vi "ActionVIOnCompile.vi"(8 "error in":errorcluster, 11 "Device Item Ref in":T16=18446744073709551615) -> (0 "error out":errorcluster)   [LabVIEW 2019, in "Fuel Injector Analysis Addon System Explorer.lvlib"]
uses:
  Fuel Injector Analysis Addon System Explorer.lvlib
  <vilib>/NI VeriStand/Custom Device API/Custom Device Item Ref.ctl
  Addon Shared/Types/Compiled.Settings.ctl
  Addon Shared/Types/Injector info.ctl
  Addon Shared/Types/Compiled.Group.WaveformRefs.ctl
  <vilib>/NI VeriStand/Custom Device API/Waveform Data Reference.ctl
  <vilib>/NI VeriStand/Custom Device API/Block Data Reference.ctl
  <vilib>/NI VeriStand/Custom Device API/Data Reference.ctl
  Addon Shared/Types/VS.Register.Info.ctl
  Addon Shared/Types/Register.Info.ctl
  Addon Shared/Types/FPGA Data Types.ctl
  Addon Shared/Types/Compiled.Group.Timing.ctl
  Addon Shared/Types/Shot.Parameters.ctl
  Addon Shared/Types/Stage.Parameters.ctl
  Addon Shared/Types/Stage.PullIn.Types.ctl
  Addon Shared/Types/Stage.Transition.Types.ctl
  Addon Shared/Types/Analysis.Channels.Select.ctl
  <vilib>/NI VeriStand/Custom Device API/Data Access Type.ctl
  <vilib>/NI VeriStand/Custom Device API/Custom Device Target Type.ctl
  Addon Shared/SubVIs/Constants.vi
  <vilib>/NI VeriStand/Custom Device Tools/Custom Device Utility Library/NI VeriStand - Search for Item by GUID.vi
  <vilib>/NI VeriStand/Custom Device Tools/Custom Device Utility Library/NI VeriStand - Search for All Items by GUID.vi
  <vilib>/NI VeriStand/Custom Device Tools/Custom Device Utility Library/NI VeriStand - Search for Item by Name.vi
  <vilib>/NI VeriStand/Custom Device API/Get Item Property (Double).vi
  <vilib>/NI VeriStand/Custom Device API/Get Item Property (U32).vi
  <vilib>/NI VeriStand/Custom Device API/Set Item Property (Variant).vi
  Addon Shared/Fuel Injector Analysis Addon Shared.lvlib
  <vilib>/NI VeriStand/Custom Device API/Custom Device API.lvlib
  <vilib>/NI VeriStand/Custom Device Tools/Custom Device Utility Library/Custom Device Utility Library.lvlib
  <vilib>/NI/NIVS Inline Async API/_Data Access System Explorer/Data Access System Explorer.lvlib
panel:
  out "output cluster":T1={"Name"="", "RIO.Address"="", "Bitfile.Path"=path "", "Injectors.Count"=0, "Injectors.Settings"=[], "Waveform.Refs"=[], "VS.Registers"={"Block Data refs"=[], "Values"=[]}, "Registers"=[], "Timing.Registers"=[], "Mux.Register"={"Name"="", "Data Type"=enum."<Null>", "Default Value"=variant(dbl 0.0)}, "Groups.Settings"=[]} {"Mux.Register"."Data Type" format="%.0x"; "Registers"."Register"."Data Type" format="%.0x"; "VS.Registers"."Block Data refs"."Data Reference" format="%.0x"}
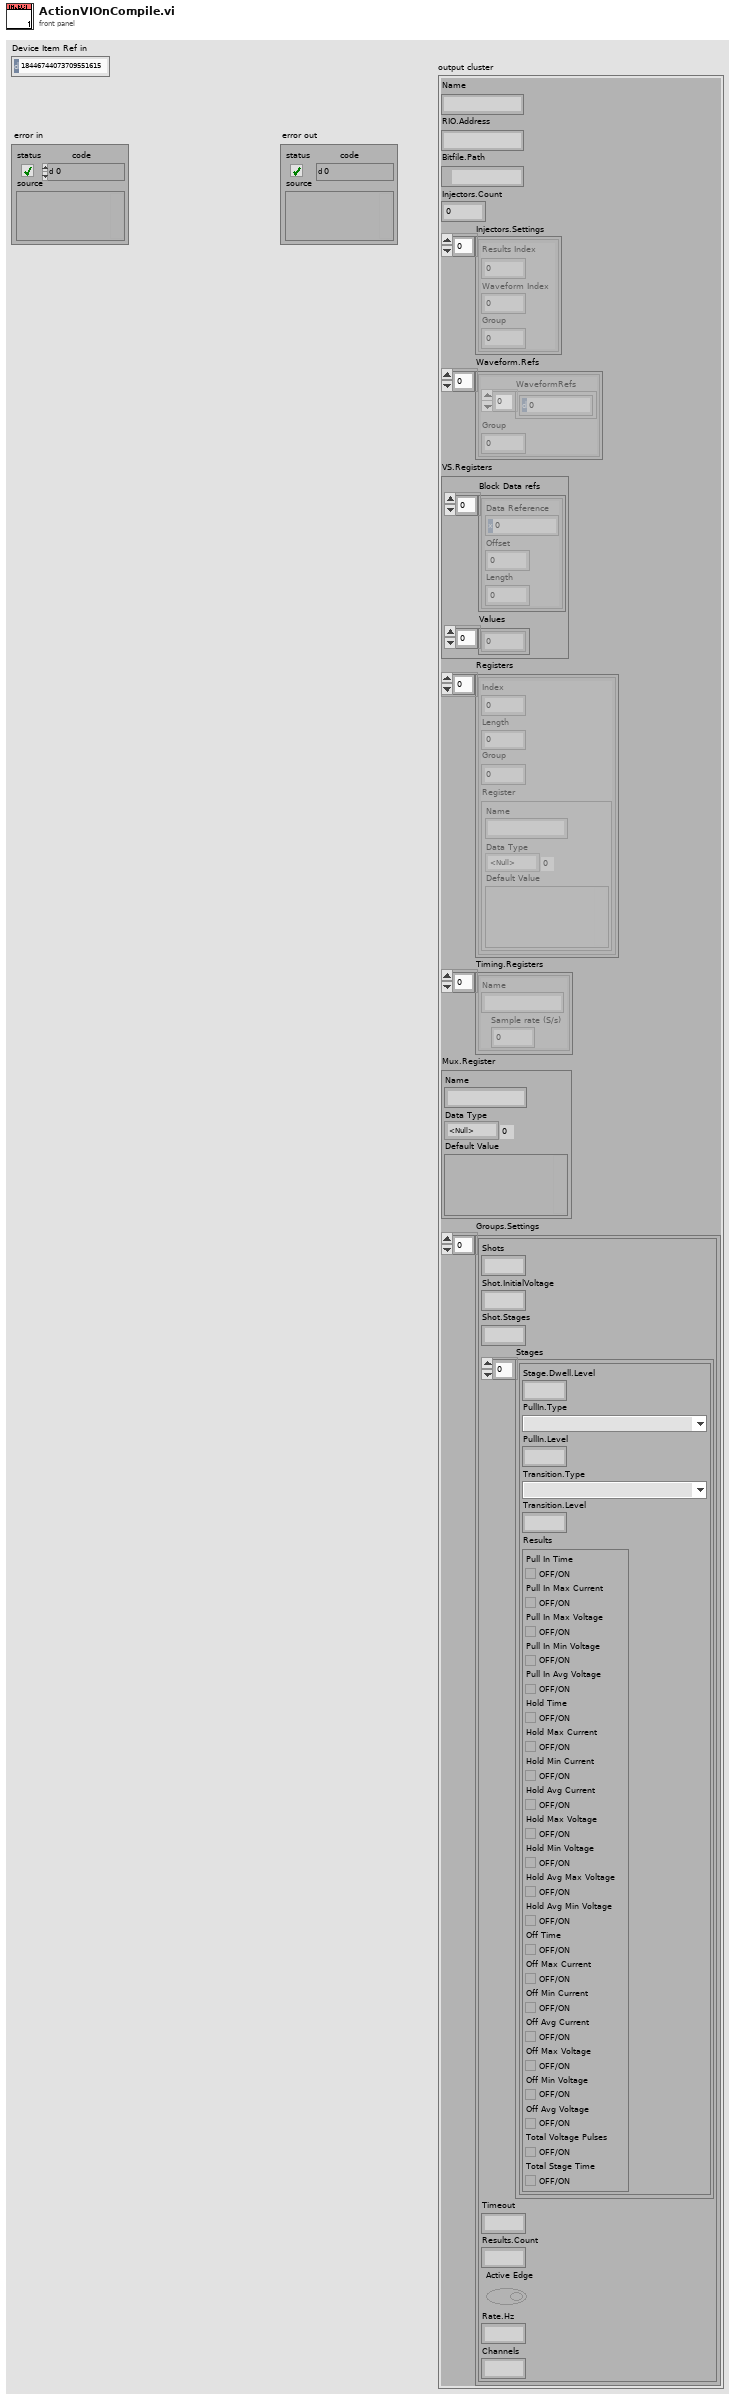
[diagram p1: front panel]
types:
  T1 = typedef "Fuel Injector Analysis Addon Shared.lvlib/Compiled.Settings.ctl" = cluster{"Name":string, "RIO.Address":string, "Bitfile.Path":path, "Injectors.Count":u32, "Injectors.Settings":T2[], "Waveform.Refs":T3[], "VS.Registers":cluster{"Block Data refs":T5[], "Values":dbl[]}, "Registers":T7[], "Timing.Registers":T10[], "Mux.Register":T8, "Groups.Settings":T11[]}
  T2 = typedef "Fuel Injector Analysis Addon Shared.lvlib/Injector info.ctl" = cluster{"Results Index":i32, "Waveform Index":i32, "Group":u16}
  T3 = typedef "Fuel Injector Analysis Addon Shared.lvlib/Compiled.Group.WaveformRefs.ctl" = cluster{"WaveformRefs":T4[], "Group":i32}
  T4 = typedef "Custom Device API.lvlib/Waveform Data Reference.ctl" = i32
  T5 = typedef "Custom Device API.lvlib/Block Data Reference.ctl" = cluster{"Data Reference":T6, "Offset":u64, "Length":u64}
  T6 = typedef "Custom Device API.lvlib/Data Reference.ctl" = i32
  T7 = typedef "Fuel Injector Analysis Addon Shared.lvlib/VS.Register.Info.ctl" = cluster{"Index":i32, "Length":i32, "Group":i32, "Register":T8}
  T8 = typedef "Fuel Injector Analysis Addon Shared.lvlib/Register.Info.ctl" = cluster{"Name":string, "Data Type":T9, "Default Value":variant}
  T9 = typedef "Fuel Injector Analysis Addon Shared.lvlib/FPGA Data Types.ctl" = enum8{"<Null>", "Injector.Core.Setting", "Injector.Global.Setting", "Injector.Mux.Setting", "Injector.Timing"}
  T10 = typedef "Fuel Injector Analysis Addon Shared.lvlib/Compiled.Group.Timing.ctl" = cluster{"Name":string, "Sample rate (S/s)":u32}
  T11 = typedef "Fuel Injector Analysis Addon Shared.lvlib/Shot.Parameters.ctl" = cluster{"Shots":u32, "Shot.InitialVoltage":dbl, "Shot.Stages":u32, "Stages":T12[], "Timeout":dbl, "Results.Count":i32, "Active Edge":bool, "Rate.Hz":u32, "Channels":u32}
  T12 = typedef "Fuel Injector Analysis Addon Shared.lvlib/Stage.Parameters.ctl" = cluster{"Stage.Dwell.Level":dbl, "PullIn.Type":T13, "PullIn.Level":dbl, "Transition.Type":T14, "Transition.Level":dbl, "Results":T15}
  T13 = typedef "Fuel Injector Analysis Addon Shared.lvlib/Stage.PullIn.Types.ctl" = enum8{"Pull In Transition Pulses", "Pull In Transition Current Drop"}
  T14 = typedef "Fuel Injector Analysis Addon Shared.lvlib/Stage.Transition.Types.ctl" = enum8{"Stage Transition Inactive Time", "Stage Transition Voltage Increase", "Stage Transition Current Decrease", "Stage Transition Active Time"}
  T15 = typedef "Fuel Injector Analysis Addon Shared.lvlib/Analysis.Channels.Select.ctl" = cluster{"Pull In Time":bool, "Pull In Max Current":bool, "Pull In Max Voltage":bool, "Pull In Min Voltage":bool, "Pull In Avg Voltage":bool, "Hold Time":bool, "Hold Max Current":bool, "Hold Min Current":bool, "Hold Avg Current":bool, "Hold Max Voltage":bool, "Hold Min Voltage":bool, "Hold Avg Max Voltage":bool, "Hold Avg Min Voltage":bool, "Off Time":bool, "Off Max Current":bool, "Off Min Current":bool, "Off Avg Current":bool, "Off Max Voltage":bool, "Off Min Voltage":bool, "Off Avg Voltage":bool, "Total Voltage Pulses":bool, "Total Stage Time":bool}
  T16 = typedef "Custom Device API.lvlib/Custom Device Item Ref.ctl" = u64
  T17 = enum16{"Output/Write", "Input/Read", "Input/ReadWrite"}
  T18 = typedef "Custom Device API.lvlib/Custom Device Target Type.ctl" = enum16{"PharLap", "VxWorks", "Windows", "Linux_32_ARM", "Linux_x64"}
  T19 = typedef "Custom Device API.lvlib/Data Access Type.ctl" = enum16{"Read", "Write"}
  T20 = cluster{"Name":string, "Type":enum16{"Output/Write", "Input/Read", "Input/ReadWrite"}, "VS Refs":T16[]}
  T21 = typedef "Custom Device API.lvlib/Custom Device Item Info.ctl" = cluster{"Name":string, "Is Channel":bool, "GUID":string, "Is Waveform":bool}
  T22 = typedef "Fuel Injector Analysis Addon Shared.lvlib/Main Settings.ctl" = cluster{"RIO Device Address":string, "Local bitfile path":path, "RT bitfile path":path, "Number of injectors":u16}
  T23 = typedef "Custom Device API.lvlib/Custom Device Channel.ctl" = cluster{"Type":T24, "Units":string, "Default Value":dbl, "Faultable":bool, "Scalable":bool}
  T24 = typedef "Custom Device API.lvlib/Custom Device Channel Type.ctl" = enum16{"Input", "Output"}
  T25 = cluster{"Name":string, "Type":enum16{"Output/Write", "Input/Read", "Input/ReadWrite"}, "VS Refs":T16[]}[]
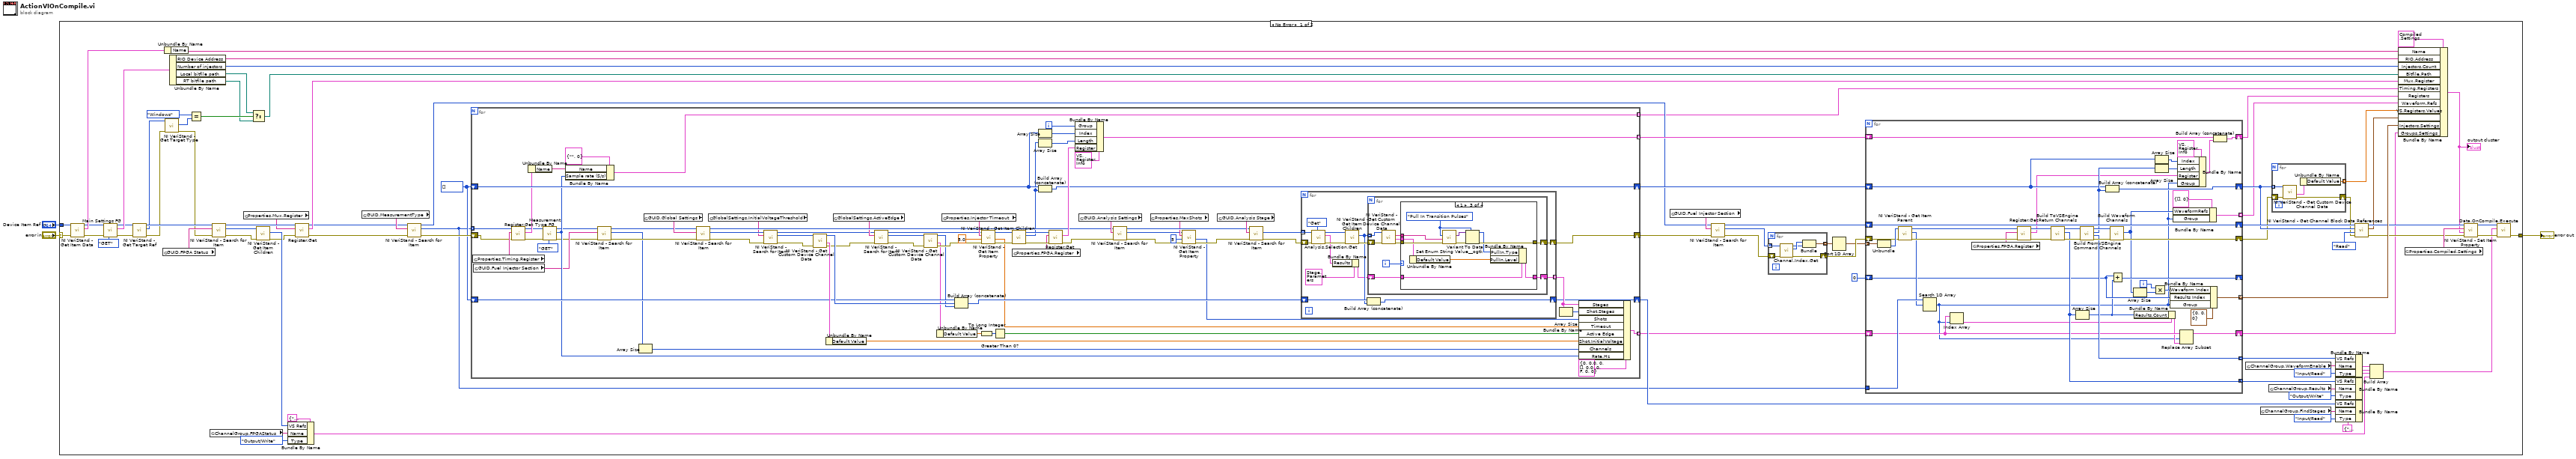
[diagram p0: block diagram]
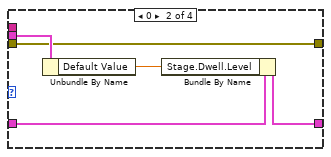
[diagram p3: hidden frame]
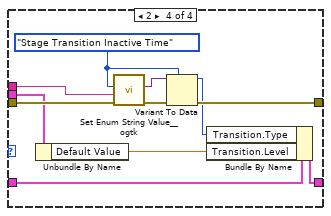
[diagram p4: hidden frame]
diagram:
  n1 = case shown="No Error" "error in" {
    selector: "error in" -> [w88 w275]
    tunnel: "Device Item Ref in" -> [w87 _]
    tunnel: [w76 w275] -> w1
    frame No Error {
      w13 = T16[] []
      w24 = T20 {"Name"="", "Type"=enum."Input/Read", "VS Refs"=[]} ("Group")
      n2 = call <vilib>:"NI VeriStand - Get Item Data.vi"("error in (no error)"=w88, "Item Ref in"=w87) -> ("error out"=w84:errorcluster, "Item Info"=w86:T21, "Item Ref out"=w83:T16)  [unwired: 6 in, 1 out]
      n3 = call "Main Settings FG.vi"("Action"=enum8{"GET", "SET"}."GET", "error in (no error)"=w84, "Item Ref"=w83) -> ("error out"=w44:errorcluster, "Main Settings out"=w82:T22, "Item Ref out"=w59:T16)  [unwired: 6 in]
      n4 = call <vilib>:"NI VeriStand - Get Target Ref.vi"("error in"=w44, "Item Ref in"=w59) -> ("error out"=w42:errorcluster, "Target Ref"=w43:T16, "Item Ref out"=w45:T16)  [unwired: 6 in, 1 out]
      n5 = global read "Constants.vi" "GUID.FPGA Status"() -> (w58:string)
      n6 = Unbundle By Name(w86) -> ("Name"=w85:string)
      n7 = call <vilib>:"NI VeriStand - Get Target Type.vi"("error in (no error)"=w42, "Item Ref in"=w43) -> ("error out"=w41:errorcluster, "Target Type"=w40:T18)  [unwired: 7 in, 1 out]
      n8 = Unbundle By Name(w82) -> ("RIO Device Address"=w81:string, "Number of injectors"=w71:u16, "Local bitfile path"=w36:path, "RT bitfile path"=w37:path)
      n9 = Equal?(x=Custom_Device_Target_Type."Windows", y=w40) -> (x = y?=w38:bool)
      n10 = global read "Constants.vi" "ChannelGroup.FPGAStatus"() -> (w55:string)
      n11 = call-poly <vilib>:"NI VeriStand - Search for Item.vi"("error in"=w41, "Item GUID"=w58, "Section Ref in"=w45) -> ("error out"=w53:errorcluster, "Item Ref"=w57:T16, "Section Ref out"=w51:T16)  [unwired: 5 in, 1 out]
      n12 = global read "Constants.vi" "Properties.Mux.Register"() -> (w49:string)
      n13 = Select(t=w36, s=w38, f=w37) -> (s? t:f=w35:path)
      n14 = call <vilib>:"NI VeriStand - Get Item Children.vi"("error in (no error)"=w53, "Item Ref in"=w57) -> ("error out"=w50:errorcluster, "Child Refs"=w54:T16[])  [unwired: 6 in, 2 out]
      n15 = Bundle By Name(cluster=T20 {"Name"="", "Type"=enum."Input/Read", "VS Refs"=[]} ("Group"), "VS Refs"=w54, "Name"=w55, "Type"=T17."Output/Write") -> (w52:T20)
      n16 = call "Register.Get.vi"("error in (no error)"=w50, "Property"=w49, "Section Ref in"=w51) -> ("error out"=w7:errorcluster, "Register"=w48:T8, "Item Ref out"=w6:T16)  [unwired: 6 in]
      n17 = global read "Constants.vi" "GUID.MeasurementType"() -> (w15:string)
      n18 = call-poly <vilib>:"NI VeriStand - Search for Item.vi"("error in"=w7, "Item GUID"=w15, "Section Ref in"=w6) -> ("error out"=w16:errorcluster, "Item Refs"=w12:T16[], "Section Ref out"=w11:T16)  [unwired: 5 in, 1 out]
      n19 = for {
        tunnel: [w126] -> w63 mode=indexing
        shift-right: [w160] -> w28
        shift-left: w16 -> [w105]
        shift-right: [w133] -> w23
        shift-left: w13 -> [w130]
        shift-right: [w124] -> w64
        shift-left: w13 -> [w128]
        tunnel: w12 -> [w104] mode=indexing
        tunnel: [w123] -> w10 mode=indexing
        tunnel: [w102] -> w5 mode=indexing
        i -> [w95]
        n20 = global read "Constants.vi" "Properties.Timing.Register"() -> (w108:string)
        n21 = global read "Constants.vi" "GUID.Fuel Injector Section"() -> (w98:string)
        n22 = call "Register.Get.vi"("error in (no error)"=w105, "Property"=w108, "Section Ref in"=w104) -> ("error out"=w94:errorcluster, "Register"=w107:T8, "Item Ref out"=w92:T16)  [unwired: 6 in]
        n23 = Unbundle By Name(w107) -> ("Name"=w106:string)
        n24 = call "Measurement Type FG.vi"("Action"=enum8{"GET", "SET"}."GET", "error in (no error)"=w94, "Item Ref"=w92) -> ("error out"=w93:errorcluster, "Sample rate (S/s)"=w101:u32, "Item Ref out"=w91:T16)  [unwired: 6 in]
        n25 = Bundle By Name(cluster=T10 {"Name"="", "Sample rate (S/s)"=0}, "Name"=w106, "Sample rate (S/s)"=w101) -> (w102:T10)
        n26 = call-poly <vilib>:"NI VeriStand - Search for Item.vi"("error in"=w93, "Item GUID"=w98, "Section Ref in"=w91) -> ("error out"=w100:errorcluster, "Item Refs"=w97:T16[], "Section Ref out"=w99:T16)  [unwired: 5 in, 1 out]
        n27 = Array Size(array=w97) -> (size(s)=w96:i32)
        n28 = global read "Constants.vi" "GUID.Global Settings"() -> (w167:string)
        n29 = call-poly <vilib>:"NI VeriStand - Search for Item.vi"("error in"=w100, "Item GUID"=w167, "Section Ref in"=w99) -> ("error out"=w141:errorcluster, "Item Ref"=w140:T16, "Section Ref out"=w149:T16)  [unwired: 5 in, 1 out]
        n30 = global read "Constants.vi" "GlobalSettings.InitialVoltageThreshold"() -> (w139:string)
        n31 = call-poly <vilib>:"NI VeriStand - Search for Item.vi"("error in"=w141, "Item Name"=w139, "Section Ref in"=w140) -> ("error out"=w136:errorcluster, "Item Ref"=w135:T16, "Section Ref out"=w118:T16)  [unwired: 5 in, 1 out]
        n32 = call <vilib>:"NI VeriStand - Get Custom Device Channel Data.vi"("error in (no error)"=w136, "Channel Ref in"=w135) -> ("error out"=w117:errorcluster, "Channel"=w137:T23, "Channel Ref out"=w134:T16)  [unwired: 4 in, 3 out]
        n33 = Unbundle By Name(w137) -> ("Default Value"=w131:dbl)
        n34 = global read "Constants.vi" "GlobalSettings.ActiveEdge"() -> (w119:string)
        n35 = call-poly <vilib>:"NI VeriStand - Search for Item.vi"("error in"=w117, "Item Name"=w119, "Section Ref in"=w118) -> ("error out"=w120:errorcluster, "Item Ref"=w121:T16, "Section Ref out"=w110:T16)  [unwired: 5 in, 1 out]
        n36 = call <vilib>:"NI VeriStand - Get Custom Device Channel Data.vi"("error in (no error)"=w120, "Channel Ref in"=w121) -> ("error out"=w116:errorcluster, "Channel"=w114:T23, "Channel Ref out"=w115:T16)  [unwired: 4 in, 3 out]
        n37 = Unbundle By Name(w114) -> ("Default Value"=w113:dbl)
        n38 = global read "Constants.vi" "Properties.Injector Timeout"() -> (w156:string)
        n39 = Build Array (concatenate)(w130, w134, w115) -> (w138:T16[])
        n40 = To Long Integer(number=w113) -> (32bit integer=w112:i32)
        n41 = call-poly <vilib>:"NI VeriStand - Get Item Property.vi"("error in (no error)"=w116, "Default Value"=5.0, "Property Name"=w156, "Item Ref in"=w110) -> ("error out"=w155:errorcluster, "Value"=w122:dbl, "Item Ref out"=w154:T16)  [unwired: 4 in, 1 out]
        n42 = Greater Than 0?(x=w112) -> (x > 0?=w111:bool)
        n43 = call <vilib>:"NI VeriStand - Get Item Children.vi"("error in (no error)"=w155, "Item Ref in"=w154) -> ("error out"=w165:errorcluster, "Child Refs"=w125:T16[], "Item Ref out"=w162:T16)  [unwired: 6 in, 1 out]
        n44 = global read "Constants.vi" "Properties.FPGA.Register"() -> (w161:string)
        n45 = Array Size(array=w128) -> (size(s)=w127:i32)
        n46 = Array Size(array=w125) -> (size(s)=w129:i32)
        n47 = Build Array (concatenate)(w128, w125) -> (w124:T16[])
        n48 = call "Register.Get.vi"("error in (no error)"=w165, "Property"=w161, "Section Ref in"=w162) -> ("error out"=w147:errorcluster, "Register"=w163:T8)  [unwired: 6 in, 1 out]
        n49 = Bundle By Name(cluster=T7 {"Index"=0, "Length"=0, "Group"=0, "Register"={"Name"="", "Data Type"=enum."<Null>", "Default Value"=variant}} ("Cluster"), "Group"=w95, "Index"=w127, "Length"=w129, "Register"=w163) -> (w126:T7)
        n50 = global read "Constants.vi" "GUID.Analysis Settings"() -> (w150:string)
        n51 = call-poly <vilib>:"NI VeriStand - Search for Item.vi"("error in"=w147, "Item GUID"=w150, "Section Ref in"=w149) -> ("error out"=w143:errorcluster, "Item Ref"=w144:T16, "Section Ref out"=w148:T16)  [unwired: 5 in, 1 out]
        n52 = global read "Constants.vi" "Properties.MaxShots"() -> (w145:string)
        n53 = call-poly <vilib>:"NI VeriStand - Get Item Property.vi"("error in (no error)"=w143, "Default Value"=u32 5, "Property Name"=w145, "Item Ref in"=w144) -> ("error out"=w142:errorcluster, "Value"=w132:u32)  [unwired: 4 in, 2 out]
        n54 = global read "Constants.vi" "GUID.Analysis Stage"() -> (w166:string)
        n55 = call-poly <vilib>:"NI VeriStand - Search for Item.vi"("error in"=w142, "Item GUID"=w166, "Section Ref in"=w148) -> ("error out"=w159:errorcluster, "Item Refs"=w158:T16[])  [unwired: 5 in, 2 out]
        n56 = for {
          tunnel: w158 -> [w180] mode=indexing
          shift-right: [w175] -> w160
          shift-left: w159 -> [w181]
          tunnel: [w174] -> w152 mode=indexing
          shift-right: [w171] -> w133
          shift-left: w138 -> [w173]
          n57 = call "Analysis.Selection.Get.vi"("Action"=enum8{"Get", "Set"}."Get", "error in (no error)"=w181, "Item Ref in"=w180) -> ("error out"=w178:errorcluster, "Selections"=w168:T15, "Item Ref out"=w176:T16)  [unwired: 6 in]
          n58 = Bundle By Name(cluster=T12 {"Stage.Dwell.Level"=0.0, "PullIn.Type"=enum."Pull In Transition Pulses", "PullIn.Level"=0.0, "Transition.Type"=enum."Stage Transition Voltage Increase", "Transition.Level"=0.0, "Results"={"Pull In Time"=TRUE, "Pull In Max Current"=TRUE, "Pull In Max Voltage"=TRUE, "Pull In Min Voltage"=TRUE, "Pull In Avg Voltage"=TRUE, "Hold Time"=TRUE, "Hold Max Current"=TRUE, "Hold Min Current"=TRUE, "Hold Avg Current"=TRUE, "Hold Max Voltage"=TRUE, "Hold Min Voltage"=TRUE, "Hold Avg Max Voltage"=TRUE, "Hold Avg Min Voltage"=TRUE, "Off Time"=TRUE, "Off Max Current"=TRUE, "Off Min Current"=TRUE, "Off Avg Current"=TRUE, "Off Max Voltage"=TRUE, "Off Min Voltage"=TRUE, "Off Avg Voltage"=TRUE, "Total Voltage Pulses"=TRUE, "Total Stage Time"=TRUE}}, "Results"=w168) -> (w169:T12)
          n59 = call <vilib>:"NI VeriStand - Get Item Children.vi"("error in (no error)"=w178, "Item Ref in"=w176) -> ("error out"=w177:errorcluster, "Child Refs"=w172:T16[])  [unwired: 6 in, 2 out]
          n60 = Build Array (concatenate)(w173, w172) -> (w171:T16[])
          n61 = for {
            shift-right: [w184] -> w175
            shift-left: w177 -> [w190]
            tunnel: w172 -> [w189] mode=indexing
            shift-right: [w182] -> w174
            shift-left: w169 -> [w183]
            i -> [w187]
            n62 = call <vilib>:"NI VeriStand - Get Custom Device Channel Data.vi"("error in (no error)"=w190, "Channel Ref in"=w189) -> ("error out"=w188:errorcluster, "Channel"=w186:T23, "Channel Name"=w185:string)  [unwired: 4 in, 3 out]
            n63 = case shown="1" w187 {
              tunnel: w188 -> [w192 w196 w208 w219]
              tunnel: w186 -> [_ w197 w203 w213]
              tunnel: w185 -> [_ _ w207 w218]
              tunnel: [w192 w196 w202 w214] -> w184
              tunnel: w183 -> [w191 w195 w201 w211]
              tunnel: [w191 w193 w200 w210] -> w182
              frame Default {
              }
              frame 0 {
                n64 = Unbundle By Name(w197) -> ("Default Value"=w194:dbl)
                n65 = Bundle By Name(cluster=w195, "Stage.Dwell.Level"=w194) -> (w193:T12)
              }
              frame 1 {
                w204 = Stage.PullIn.Types."Pull In Transition Pulses" ("PullIn.Type")
                n66 = Unbundle By Name(w203) -> ("Default Value"=w198:dbl)
                n67 = call <userlib>:"Set Enum String Value__ogtk.vi"("error in (no error)"=w208, "String Value"=w207, "Default Enum Value"=w204) -> ("error out"=w206:errorcluster, "Enum"=w205:variant)  [unwired: 7 in]
                n68 = Variant To Data(error in=w206, type=w204, Variant=w205) -> (data=w199:T13, error out=w202:errorcluster)
                n69 = Bundle By Name(cluster=w201, "PullIn.Type"=w199, "PullIn.Level"=w198) -> (w200:T12)
              }
              frame 2 {
                w215 = Stage.Transition.Types."Stage Transition Inactive Time" ("Stage.Transition")
                n70 = Unbundle By Name(w213) -> ("Default Value"=w212:dbl)
                n71 = call <userlib>:"Set Enum String Value__ogtk.vi"("error in (no error)"=w219, "String Value"=w218, "Default Enum Value"=w215) -> ("error out"=w217:errorcluster, "Enum"=w216:variant)  [unwired: 7 in]
                n72 = Variant To Data(error in=w217, type=w215, Variant=w216) -> (data=w209:T14, error out=w214:errorcluster)
                n73 = Bundle By Name(cluster=w211, "Transition.Type"=w209, "Transition.Level"=w212) -> (w210:T12)
              }
            }
          }
        }
        n74 = Array Size(array=w152) -> (size(s)=w151:i32)
        n75 = Bundle By Name(cluster=T11 {"Shots"=0, "Shot.InitialVoltage"=0.0, "Shot.Stages"=0, "Stages"=[], "Timeout"=0.0, "Results.Count"=0, "Active Edge"=FALSE, "Rate.Hz"=0, "Channels"=0} ("Parameters"), "Stages"=w152, "Shot.Stages"=w151, "Shots"=w132, "Timeout"=w122, "Active Edge"=w111, "Shot.InitialVoltage"=w131, "Channels"=w96, "Rate.Hz"=w101) -> (w123:T11)
      }
      n76 = global read "Constants.vi" "GUID.Fuel Injector Section"() -> (w80:string)
      n77 = call-poly <vilib>:"NI VeriStand - Search for Item.vi"("error in"=w28, "Item GUID"=w80, "Section Ref in"=w11) -> ("error out"=w20:errorcluster, "Item Refs"=w21:T16[], "Section Ref out"=w79:T16)  [unwired: 5 in, 1 out]
      n78 = for {
        tunnel: w21 -> [w225] mode=indexing
        shift-right: [w223] -> w19
        shift-left: w20 -> [w224]
        tunnel: [w220] -> w18 mode=indexing
        n79 = call "Channel.Index.Get.vi"("error in (no error)"=w224, "Ref in"=w225) -> ("error out"=w223:errorcluster, "Value"=w222:u16, "Ref out"=w221:T16)  [unwired: 6 in, 1 out]
        n80 = Bundle("Value"=w222, "Ref out"=w221) -> (w220:cluster{"Value":u16, "Ref out":T16})  [unwired: 1 in]
      }
      n81 = Sort 1D Array(array=w18) -> (sorted array=w17:cluster{"Value":u16, "Ref out":T16}[])
      n82 = for {
        shift-right: [w267] -> w30
        shift-left: w19 -> [w242]
        tunnel: [w257] -> w72 mode=indexing
        shift-right: [w266] -> w46
        shift-left: w79 -> [w266]
        tunnel: [w263] -> w70 mode=concatenating
        tunnel: [w259] -> w69 mode=indexing
        shift-right: [w250] -> w32
        shift-left: w64 -> [w251]
        shift-right: [w249] -> w60
        shift-left: w63 -> [w254]
        tunnel: w17 -> [w245] mode=indexing
        tunnel: w12 -> [w240]
        shift-right: [w234] -> w14
        shift-left: w10 -> [w236]
        shift-right: [w230] -> _
        shift-left: 0 -> [w232]
        tunnel: [w227] -> w4 mode=indexing
        i -> [w262]
        n83 = Unbundle(w245) -> ("Ref out"=w244:T16)  [unwired: 1 out]
        n84 = call <vilib>:"NI VeriStand - Get Item Parent.vi"("error in (no error)"=w242, "Item Ref in"=w244) -> ("error out"=w241:errorcluster, "Parent Ref"=w239:T16, "Item Ref out"=w243:T16)  [unwired: 6 in, 1 out]
        n85 = Search 1D Array(1D array=w240, element=w239) -> (index of element=w226:i32)  [unwired: 1 in]
        n86 = Index Array(array=w236, index=w226) -> (element=w238:T11)
        n87 = global read "Constants.vi" "Properties.FPGA.Register"() -> (w237:string)
        n88 = call "Register.Get.vi"("error in (no error)"=w241, "Property"=w237, "Section Ref in"=w243) -> ("error out"=w248:errorcluster, "Register"=w246:T8, "Item Ref out"=w247:T16)  [unwired: 6 in]
        n89 = call "Build ToVSEngine Return Channels.vi"("error in (no error)"=w248, "Injector section ref in"=w247) -> ("error out"=w269:errorcluster, "Results"=w263:T16[], "Injector section ref out"=w264:T16)  [unwired: 7 in]
        n90 = Array Size(array=w263) -> (size(s)=w231:i32)
        n91 = call "Build FromVSEngine Command Channels.vi"("error in (no error)"=w269, "Injector section ref in"=w264) -> ("error out"=w268:errorcluster, "WaveformEnable?"=w257:T16, "InjectionSettings"=w252:T16[], "Injector section ref out"=w258:T16)  [unwired: 6 in]
        n92 = Build Array (concatenate)(w251, w252) -> (w250:T16[])
        n93 = call "Build Waveform Channels.vi"("error in (no error)"=w268, "Injector section ref in"=w258) -> ("error out"=w267:errorcluster, "Waveform channel array out"=w229:T4[])  [unwired: 7 in, 1 out]
        n94 = Add(x=w232, y=w231) -> (x+y=w230:i32)
        n95 = Array Size(array=w229) -> (size(s)=w265:i32)
        n96 = Bundle By Name(cluster=w238, "Results.Count"=w231) -> (w235:T11)
        n97 = Multiply(x=w262, y=w265) -> (x*y=w260:i32)
        n98 = Array Size(array=w251) -> (size(s)=w255:i32)
        n99 = Array Size(array=w252) -> (size(s)=w233:i32)
        n100 = Bundle By Name(cluster=T2 {"Results Index"=0, "Waveform Index"=0, "Group"=0} ("Injector info"), "Waveform Index"=w260, "Results Index"=w232, "Group"=w226) -> (w259:T2)
        n101 = Bundle By Name(cluster=T3 {"WaveformRefs"=[], "Group"=0}, "WaveformRefs"=w229, "Group"=w226) -> (w227:T3)
        n102 = Bundle By Name(cluster=T7 {"Index"=0, "Length"=0, "Group"=0, "Register"={"Name"="", "Data Type"=enum."<Null>", "Default Value"=variant}} ("Cluster"), "Index"=w255, "Length"=w233, "Register"=w246, "Group"=w226) -> (w253:T7)
        n103 = Replace Array Subset(array=w236, new element=w235, index=w226) -> (w234:T11[])
        n104 = Build Array (concatenate)(w254, w253) -> (w249:T7[])
      }
      n105 = global read "Constants.vi" "ChannelGroup.WaveformEnable"() -> (w73:string)
      n106 = global read "Constants.vi" "ChannelGroup.FindStages"() -> (w25:string)
      n107 = global read "Constants.vi" "ChannelGroup.Results"() -> (w74:string)
      n108 = for {
        tunnel: w32 -> [w274] mode=indexing
        shift-right: [w272] -> w29
        shift-left: w30 -> [w273]
        tunnel: [w270] -> w31 mode=indexing
        n109 = call <vilib>:"NI VeriStand - Get Custom Device Channel Data.vi"("error in (no error)"=w273, "Channel Ref in"=w274) -> ("error out"=w272:errorcluster, "Channel"=w271:T23)  [unwired: 4 in, 4 out]
        n110 = Unbundle By Name(w271) -> ("Default Value"=w270:dbl)
      }
      n111 = Bundle By Name(cluster=w24, "VS Refs"=w72, "Name"=w73, "Type"=T17."Input/Read") -> (w67:T20)
      n112 = Bundle By Name(cluster=w24, "VS Refs"=w70, "Name"=w74, "Type"=T17."Output/Write") -> (w68:T20)
      n113 = Bundle By Name(cluster=w24, "VS Refs"=w23, "Name"=w25, "Type"=T17."Input/Read") -> (w22:T20)
      n114 = call <vilib>:"NI VeriStand - Get Channel Block Data References.vi"("error in (no error)"=w29, "Access"=Data_Access_Type."Read", "Channel Refs"=w32, "Device Ref in"=w46) -> ("error out"=w61:errorcluster, "Block Data Refs"=w9:T5[], "Device Ref out"=w47:T16)  [unwired: 4 in, 1 out]
      n115 = Build Array(w67, w68, w22, w52) -> (w33:T25)
      n116 = Bundle By Name(cluster=T1 {"Name"="", "RIO.Address"="", "Bitfile.Path"=path "", "Injectors.Count"=0, "Injectors.Settings"=[], "Waveform.Refs"=[], "VS.Registers"={"Block Data refs"=[], "Values"=[]}, "Registers"=[], "Timing.Registers"=[], "Mux.Register"={"Name"="", "Data Type"=enum."<Null>", "Default Value"=variant(dbl 0.0)}, "Groups.Settings"=[]} ("Settings.Compiled"), "Name"=w85, "RIO.Address"=w81, "Injectors.Count"=w71, "Bitfile.Path"=w35, "Mux.Register"=w48, "Timing.Registers"=w5, "Registers"=w60, "Waveform.Refs"=w4, "VS.Registers.Values"=w31, "VS.Registers.Block Data refs"=w9, "Injectors.Settings"=w69, "Groups.Settings"=w14) -> (w34:T1)
      "output cluster" <- w34
      n117 = global read "Constants.vi" "Properties.Compiled.Settings"() -> (w90:string)
      n118 = call-poly <vilib>:"NI VeriStand - Set Item Property.vi"("error in (no error)"=w61, "Value"=w34, "Property Name"=w90, "Item Ref in"=w47) -> ("error out"=w77:errorcluster, "Item Ref out"=w75:T16)  [unwired: 5 in, 1 out]
      n119 = call <vilib>:"Data.OnCompile.Execute.vi"("error in"=w77, "VS Ref Groups"=w33, "Custom Device Ref"=w75) -> ("error out"=w76:errorcluster)  [unwired: 7 in, 1 out]
    }
    frame Error {
    }
  }
  "error out" <- w1
